vi "niRFUtil MASMT 1D FFT (CDB).vi"(0 "X":cdb[](array[numeric]), 1 "shift?":bool, 5 "FFT size":i32=-1, 11 "error in (no error)":errorcluster) -> (4 "FFT {X}":cdb[](array[numeric]), 15 "error out":errorcluster)   [LabVIEW 2015, in "niRFUtil.lvlib"]
doc: "Computes the fast Fourier transform (FFT) of the input sequence <B>X</B>."
uses:
  niRFUtil.lvlib
  Utilities/niRFMASMT_FFT.dll
panel:
  out "Workspace":cdb[](array[numeric])
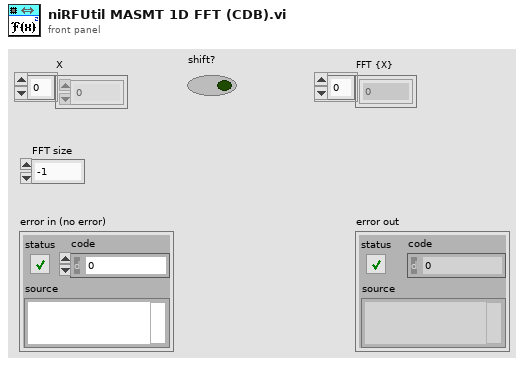
[diagram p1: front panel]
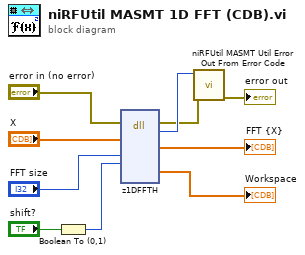
[diagram p0: block diagram]
diagram:
  n1 = Boolean To (0,1)(Boolean="shift?") -> (0, 1=w5:i16)
  n2 = dll-call lib="C:/Perforce/semoore-sales/Customers/NATI-3813/Noise Floor/LV Filters/ParallelComplexFilterRFUtil/niRFUtil/MASMT/Utilities/niRFMASMT_FFT.*" fn="z1DFFTH" ("lvanlys.dll:ReNIFFTH80")(error in="error in (no error)", "xH"="X", "fftSize"="FFT size", "shift"=w5) -> (error out=w1:errorcluster, "return type"=w4:i32, "FFT {X}"=→"FFT {X}":cdb[], "Workspace"=→"Workspace":cdb[])  [unwired: 9 in, 1 out]
  n3 = call "niRFUtil MASMT Util Error Out From Error Code.vi"("error in (no error)"=w1, "error code"=w4) -> ("error out"=→"error out":errorcluster)  [unwired: 9 in]
